vi "Stop Device.vi"(8 "error in":errorcluster, 11 "CnPt in":refnum<class "CnPt.lvclass">) -> (0 "error out":errorcluster, 3 "CnPt out":refnum<class "CnPt.lvclass">)   [LabVIEW 2015, in "CnPt.lvclass"]
uses:
  CnPt.lvclass
  <vilib>/MSR Consulting, LLC/General Reuse/Session APIs/Serial/Serial Session.lvclass
  CnPt.lvclass/CnPt.ctl
  <vilib>/MSR Consulting, LLC/Devices/Configurable Device/Configurable Device.lvclass
  <vilib>/MSR Consulting, LLC/General Reuse/Session APIs/_Session Fwk/Session - Root.lvclass
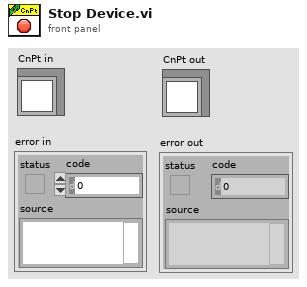
[diagram p1: front panel]
types:
  T1 = typedef "Serial Session.lvclass/Session Handle.ctl" = refnum<data-value>
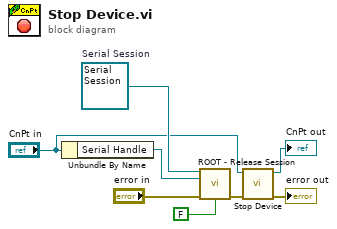
[diagram p0: block diagram]
diagram:
  w4 = refnum<class "Serial Session.lvclass"> refnum  # Serial Session
  n1 = Unbundle By Name("CnPt in") -> ("Serial Handle"=w6:T1)
  n2 = call <vilib>:"ROOT - Release Session.vi"("OBJ - Session in"=w4, "Session Handle in"=w6, "error in (no error)"="error in", "force destroy? (F)"=FALSE) -> ("error out"=w2:errorcluster)  [unwired: 10 in, 1 out]
  n3 = call-parent "Stop Device.vi"("error in"=w2, "Configurable Device in"="CnPt in") -> ("error out"=→"error out":errorcluster, "Configurable Device out"=→"CnPt out":refnum<class "CnPt.lvclass">)  [unwired: 8 in]
